vi "AIN EF Config Tool for build.vi"() -> (0 "error out":errorcluster)   [LabVIEW 2020]
panel:
  out "# Config Reads":i32
  in  "Read Config":bool
  in  "Set Defaults":bool
  out "# Reads":i32
  in  "Read Values":bool
  out "Names Read":string[](array[string])
  out "Read Values":dbl[](array[numeric]) format="%.6f"
  in  "Generic Names for Reads":string[](array[string])=["AIN#(0:254)_EF_READ_A", "AIN#(0:254)_EF_READ_B", "AIN#(0:254)_EF_READ_C", "AIN#(0:254)_EF_READ_D"]
  in  "Exit":bool
  out "# Config Writes":i32
  in  "Write Config":bool
  out "Config Names":string[](array[string])
  in  "Channel #":i32
  out "Error String":string="No Error"
  out "ConnectionType Out":i32
  out "DeviceType Out":i32
  in  "Identifier":string="LJM_idANY"
  in  "ConnectionType":string="LJM_ctANY"
  in  "DeviceType":string="LJM_dtANY"
  in  "Config Values":dbl[](array[numeric])=[0.0, 0.0, 0.0, 0.0, 0.0, 0.0, 0.0, 0.0, 0.0, 0.0, 0.0, 10.0, 199.0, 0.0] format="%.9f"
  in  "Generic Names for Config":string[](array[string])=["AIN#(0:254)_EF_INDEX", "AIN#(0:254)_EF_CONFIG_A", "AIN#(0:254)_EF_CONFIG_B", "AIN#(0:254)_EF_CONFIG_C", "AIN#(0:254)_EF_CONFIG_D", "AIN#(0:254)_EF_CONFIG_E", "AIN#(0:254)_EF_CONFIG_F", "AIN#(0:254)_EF_CONFIG_G", "AIN#(0:254)_EF_CONFIG_H", "AIN#(0:254)_EF_CONFIG_I", "AIN#(0:254)_EF_CONFIG_J", "AIN#(0:254)_RANGE", "AIN#(0:254)_NEGATIVE_CH", "AIN#(0:254)_RESOLUTION_INDEX"]
  out "ErrorAddress":i32
  # "When you click \"Write Config\" or \"Read Values\", this program does open-write-read-close.  That means that in between a write or read you can run another program such as Kipling or LJLogM."
  # "Writes a 1 to IO_CONFIG_SET_DEFAULT_TO_CURRENT.\nTakes the current status of the entire IO Config system\nand saves it as the reboot default.  See:\nhttp://labjack.com/support/datasheets/t-series/io-config-default"
  # "See the AIN-EF documentation:\n\nhttps://labjack.com/support/datasheets/t-series/ain/extended-features"
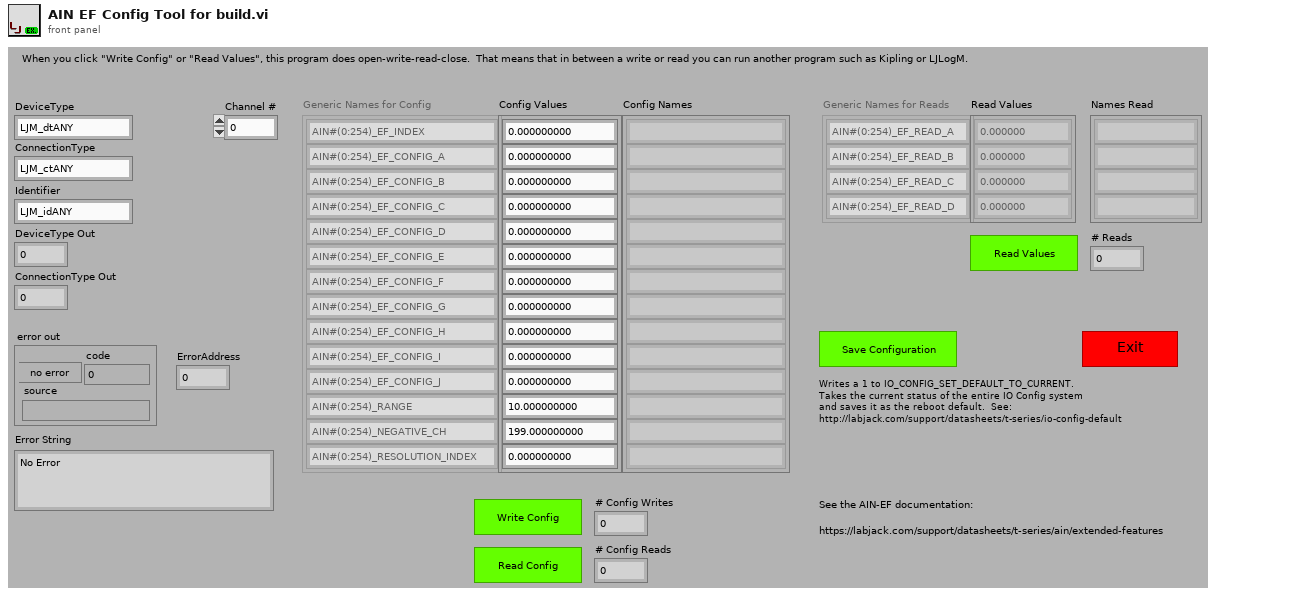
[diagram p1: front panel]
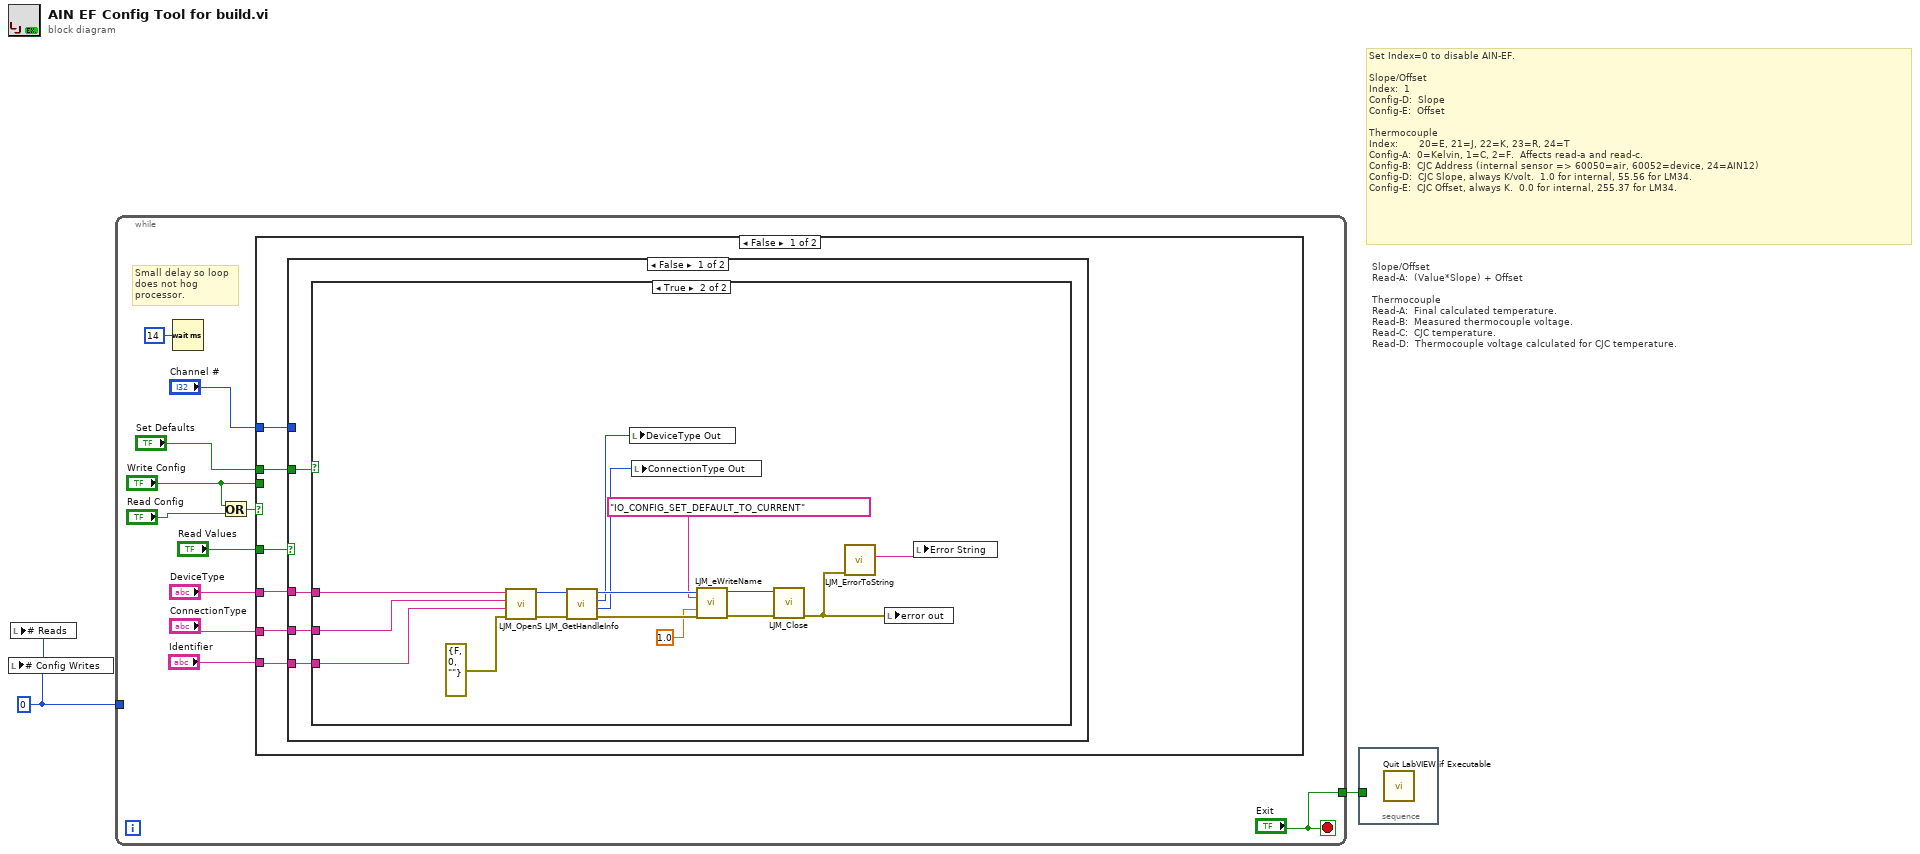
[diagram p0: block diagram]
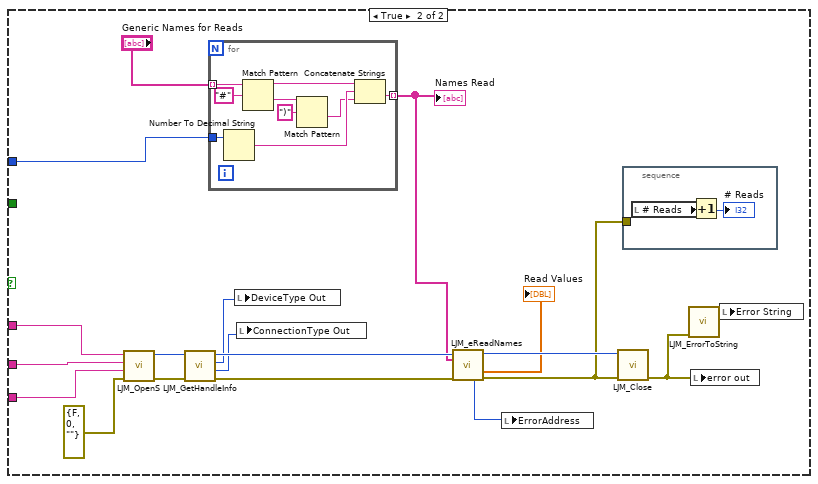
[diagram p3: hidden frame]
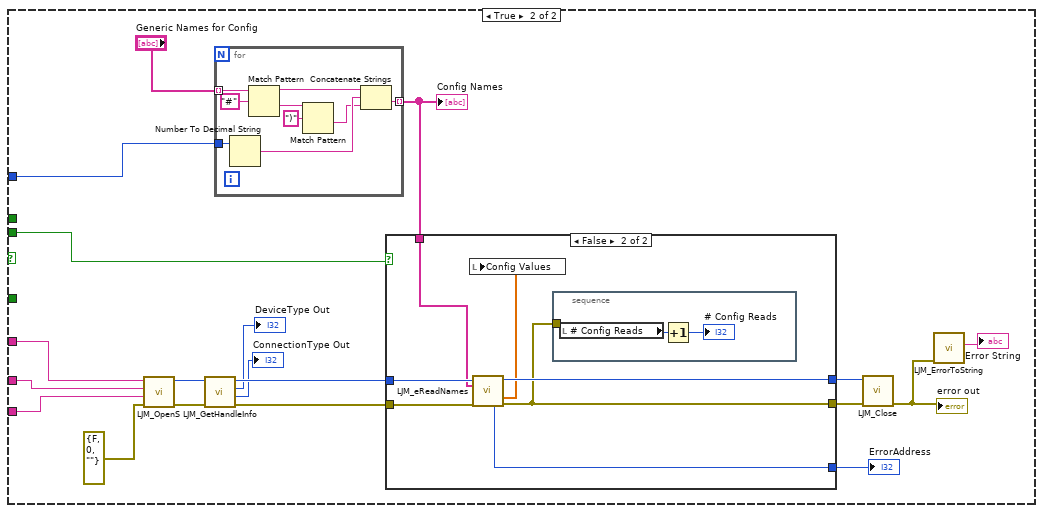
[diagram p4: hidden frame]
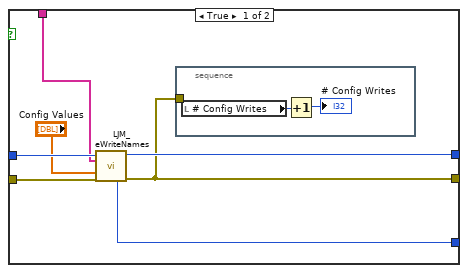
[diagram p5: hidden frame]
diagram:
  w1 = 0 ("# Writes")
  # "Slope/Offset\nRead-A:  (Value*Slope) + Offset\n\nThermocouple\nRead-A:  Final calculated temperature.\nRead-B:  Measured thermocouple voltage.\nRead-C:  CJC temperature.\nRead-D:  Thermocouple voltage calculated for CJC temperature."
  # "Set Index=0 to disable AIN-EF.\n\nSlope/Offset\nIndex:  1\nConfig-D:  Slope\nConfig-E:  Offset\n\nThermocouple\nIndex:       20=E, 21=J, 22=K, 23=R, 24=T\nConfig-A:  0=Kelvin, 1=C, 2=F.  Affects read-a and read-c.\nConfig-B:  CJC Address (internal sensor => 60050=air, 60052=device, 24=AIN12)\nConfig-D:  CJC Slope, always K/volt.  1.0 for internal, 55.56 for LM34.\nConfig-E:  CJC Offset, always K.  0.0 for internal, 255.37 for LM34."
  n1 = local write "# Config Writes"(w1) -> ()
  n2 = local write "# Reads"(w1) -> ()
  n3 = while {
    tunnel: w1 -> [_]
    tunnel: ["Exit"] -> w2
    stop <- "Exit" stop-if-true
    # "Small delay so loop\ndoes not hog\nprocessor."
    n4 = Wait (ms)(milliseconds to wait=u32 14) -> ()  [unwired: 1 out]
    n5 = Or(x="Write Config", y="Read Config") -> (x .or. y?=w5:bool)
    n6 = case shown="False" w5 {
      tunnel: "Read Values" -> [w19 _]
      tunnel: "Identifier" -> [w18 w75]
      tunnel: "ConnectionType" -> [w17 w74]
      tunnel: "DeviceType" -> [w16 w73]
      tunnel: "Channel #" -> [w15 w72]
      tunnel: "Set Defaults" -> [w14 _]
      tunnel: "Write Config" -> [_ w70]
      frame False {
        n7 = case shown="False" w19 {
          tunnel: w18 -> [w20 w47]
          tunnel: w17 -> [w21 w46]
          tunnel: w16 -> [w22 w45]
          tunnel: w15 -> [_ w41]
          tunnel: w14 -> [w23 _]
          frame False {
            n8 = case shown="True" w23 {
              tunnel: w22 -> [_ w32]
              tunnel: w21 -> [_ w31]
              tunnel: w20 -> [_ w30]
              frame False {
              }
              frame True {
                n9 = call "LJM_OpenS.vi"("error in"=errorcluster {"status"=FALSE, "code"=0, "source"=""} ("error in (no error)"), "Identifier"=w30, "ConnectionType"=w31, "DeviceType"=w32) -> ("error out"=w38:errorcluster, "Handle"=w36:i32)  [unwired: 6 in]
                n10 = call "LJM_GetHandleInfo.vi"("error in"=w38, "Handle In"=w36) -> ("error out"=w37:errorcluster, "ConnectionType"=w28:i32, "DeviceType"=w29:i32, "Handle Out"=w35:i32)  [unwired: 2 in, 4 out]
                n11 = local write "DeviceType Out"(w29) -> ()
                n12 = local write "ConnectionType Out"(w28) -> ()
                n13 = call "LJM_eWriteName.vi"("Handle In"=w35, "Name"="IO_CONFIG_SET_DEFAULT_TO_CURRENT", "Value"=1.0, "error in"=w37) -> ("Handle Out"=w34:i32, "error out"=w33:errorcluster)  [unwired: 10 in]
                n14 = call "LJM_Close.vi"("error in"=w33, "Handle"=w34) -> ("error out"=w25:errorcluster)  [unwired: 9 in]
                n15 = call "LJM_ErrorToString.vi"("error in"=w25) -> ("String"=w24:string)  [unwired: 10 in]
                n16 = local write "error out"(w25) -> ()
                n17 = local write "Error String"(w24) -> ()
              }
            }
          }
          frame True {
            n18 = call "LJM_OpenS.vi"("error in"=errorcluster {"status"=FALSE, "code"=0, "source"=""} ("error in (no error)"), "Identifier"=w47, "ConnectionType"=w46, "DeviceType"=w45) -> ("error out"=w54:errorcluster, "Handle"=w56:i32)  [unwired: 6 in]
            n19 = call "LJM_GetHandleInfo.vi"("error in"=w54, "Handle In"=w56) -> ("error out"=w55:errorcluster, "ConnectionType"=w42:i32, "DeviceType"=w43:i32, "Handle Out"=w57:i32)  [unwired: 2 in, 4 out]
            n20 = for {
              tunnel: "Generic Names for Reads" -> [w69] mode=indexing
              tunnel: w41 -> [w64]
              tunnel: [w61] -> w52 mode=indexing
              n21 = Number To Decimal String(number=w64) -> (decimal integer string=w63:string)  [unwired: 1 in]
              n22 = Match Pattern(string=w69, regular expression="#") -> (before substring=w65:string, after substring=w67:string)  [unwired: 1 in, 2 out]
              n23 = Match Pattern(string=w67, regular expression=")") -> (after substring=w62:string)  [unwired: 1 in, 3 out]
              n24 = Concatenate Strings(w65, w63, w62) -> (w61:string)
            }
            "Names Read" <- w52
            n25 = local write "DeviceType Out"(w43) -> ()
            n26 = local write "ConnectionType Out"(w42) -> ()
            n27 = call "LJM_eReadNames.vi"("Handle In"=w57, "aNames"=w52, "error in"=w55) -> ("Handle Out"=w58:i32, "aValuesOut"=→"Read Values":dbl[], "ErrorAddress"=w51:i32, "error out"=w40:errorcluster)  [unwired: 9 in]
            n28 = local write "ErrorAddress"(w51) -> ()
            n29 = call "LJM_Close.vi"("error in"=w40, "Handle"=w58) -> ("error out"=w50:errorcluster)  [unwired: 9 in]
            n30 = stacked-sequence {
              tunnel: w40 -> [_]
              frame #0 {
                n31 = local read "# Reads"() -> (w59:i32)
                n32 = Increment(x=w59) -> (x+1=→"# Reads":i32)
              }
            }
            n33 = call "LJM_ErrorToString.vi"("error in"=w50) -> ("String"=w49:string)  [unwired: 10 in]
            n34 = local write "error out"(w50) -> ()
            n35 = local write "Error String"(w49) -> ()
          }
        }
      }
      frame True {
        n36 = call "LJM_OpenS.vi"("error in"=errorcluster {"status"=FALSE, "code"=0, "source"=""} ("error in (no error)"), "Identifier"=w75, "ConnectionType"=w74, "DeviceType"=w73) -> ("error out"=w87:errorcluster, "Handle"=w85:i32)  [unwired: 6 in]
        n37 = call "LJM_GetHandleInfo.vi"("error in"=w87, "Handle In"=w85) -> ("error out"=w86:errorcluster, "ConnectionType"=→"ConnectionType Out":i32, "DeviceType"=→"DeviceType Out":i32, "Handle Out"=w84:i32)  [unwired: 2 in, 4 out]
        n38 = for {
          tunnel: "Generic Names for Config" -> [w115] mode=indexing
          tunnel: w72 -> [w110]
          tunnel: [w107] -> w76 mode=indexing
          n39 = Number To Decimal String(number=w110) -> (decimal integer string=w109:string)  [unwired: 1 in]
          n40 = Match Pattern(string=w115, regular expression="#") -> (before substring=w111:string, after substring=w113:string)  [unwired: 1 in, 2 out]
          n41 = Match Pattern(string=w113, regular expression=")") -> (after substring=w108:string)  [unwired: 1 in, 3 out]
          n42 = Concatenate Strings(w111, w109, w108) -> (w107:string)
        }
        "Config Names" <- w76
        n43 = case shown="False" w70 {
          tunnel: w86 -> [w95 w104]
          tunnel: w84 -> [w94 w103]
          tunnel: [w93 w102] -> w83
          tunnel: [w92 w101] -> w79
          tunnel: w76 -> [w90 w100]
          tunnel: [w89 w99] -> w71
          frame True {
            n44 = call "LJM_eWriteNames.vi"("Handle In"=w94, "aNames"=w90, "aValuesIn"="Config Values", "error in"=w95) -> ("Handle Out"=w93:i32, "ErrorAddress"=w92:i32, "error out"=w89:errorcluster)  [unwired: 9 in]
            n45 = stacked-sequence {
              tunnel: w89 -> [_]
              frame #0 {
                n46 = local read "# Config Writes"() -> (w97:i32)
                n47 = Increment(x=w97) -> (x+1=→"# Config Writes":i32)
              }
            }
          }
          frame False {
            n48 = call "LJM_eReadNames.vi"("Handle In"=w103, "aNames"=w100, "error in"=w104) -> ("Handle Out"=w102:i32, "aValuesOut"=w98:dbl[], "ErrorAddress"=w101:i32, "error out"=w99:errorcluster)  [unwired: 9 in]
            n49 = local write "Config Values"(w98) -> ()
            n50 = stacked-sequence {
              tunnel: w99 -> [_]
              frame #0 {
                n51 = local read "# Config Reads"() -> (w105:i32)
                n52 = Increment(x=w105) -> (x+1=→"# Config Reads":i32)
              }
            }
          }
        }
        "ErrorAddress" <- w79
        n53 = call "LJM_Close.vi"("error in"=w71, "Handle"=w83) -> ("error out"=w80:errorcluster)  [unwired: 9 in]
        "error out" <- w80
        n54 = call "LJM_ErrorToString.vi"("error in"=w80) -> ("String"=→"Error String":string)  [unwired: 10 in]
      }
    }
  }
  n55 = stacked-sequence {
    tunnel: w2 -> [_]
    frame #0 {
      n56 = call "Quit LabVIEW if Executable.vi"() -> ()  [unwired: 1 in]
    }
  }
